vi "Core Actor - INIT - External Queues_Notifiers.vi"(8 "error in (no error)":errorcluster, 11 "Child_1_Class in":refnum<class "GUI_Class.lvclass">) -> (0 "error out":errorcluster, 3 "Child_1_Class out":refnum<class "GUI_Class.lvclass">)   [LabVIEW 2023, in "GUI_Actor.lvlib" / "GUI_Class.lvclass"]
uses:
  GUI_Class.lvclass
  GUI_Class.lvclass/GUI_Class.ctl
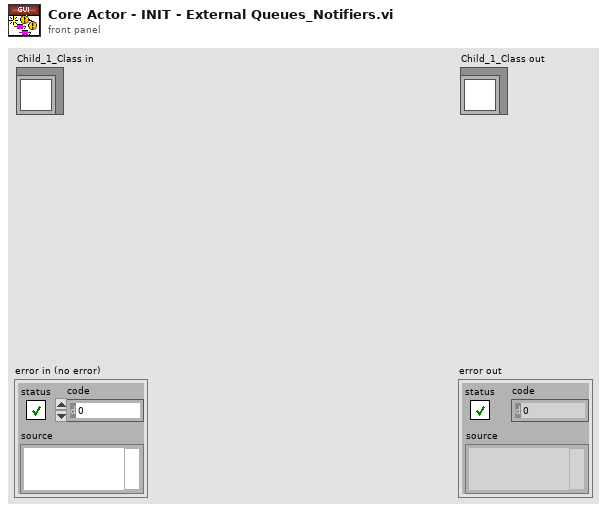
[diagram p1: front panel]
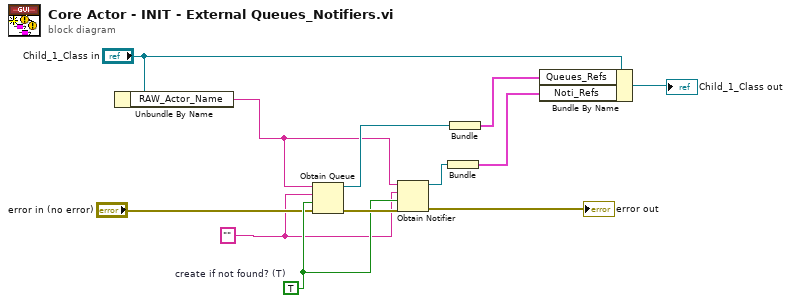
[diagram p0: block diagram]
diagram:
  w4 = ""
  w10 = TRUE  # create if not found? (T)
  n1 = Unbundle By Name("Child_1_Class in") -> ("RAW_Actor_Name"=w5:string)
  n2 = Obtain Queue(name (unnamed)=w5, element data type=w4, create if not found? (T)=w10, error in (no error)="error in (no error)") -> (queue out=w9:refnum<queue>, error out=w11:errorcluster)  [unwired: 1 in, 1 out]
  n3 = Obtain Notifier(name (unnamed)=w5, notification data type=w4, create if not found? (T)=w10, error in (no error)=w11) -> (notifier out=w8:refnum<notifier>, error out=→"error out":errorcluster)  [unwired: 1 out]
  n4 = Bundle("notifier out"=w8) -> (w2:cluster{"notifier out":refnum<notifier>})  [unwired: 1 in]
  n5 = Bundle("queue out"=w9) -> (w3:cluster{"queue out":refnum<queue>})  [unwired: 1 in]
  n6 = Bundle By Name(cluster="Child_1_Class in", "Queues_Refs"=w3, "Noti_Refs"=w2) -> (→"Child_1_Class out":refnum<class "GUI_Class.lvclass">)
